vi "lab8.1.vi"() -> ()   [LabVIEW 2018]
panel:
  out "#":dbl
  in  "SELECTOR":sgl(knob) scale=0.0..2.0 scale format="%#_1g"
  out "#3":dbl format="%#_1g"
  out "#2":dbl format="%#_1g"
  out "#1":dbl format="%#_1g"
  in  "PRESS TO\nROLL":bool
  out "output\nnumber":dbl
  in  "toggle":bool
  # "10 & 20\nTOGGLE"
  # "RANDOM #\nGEN"
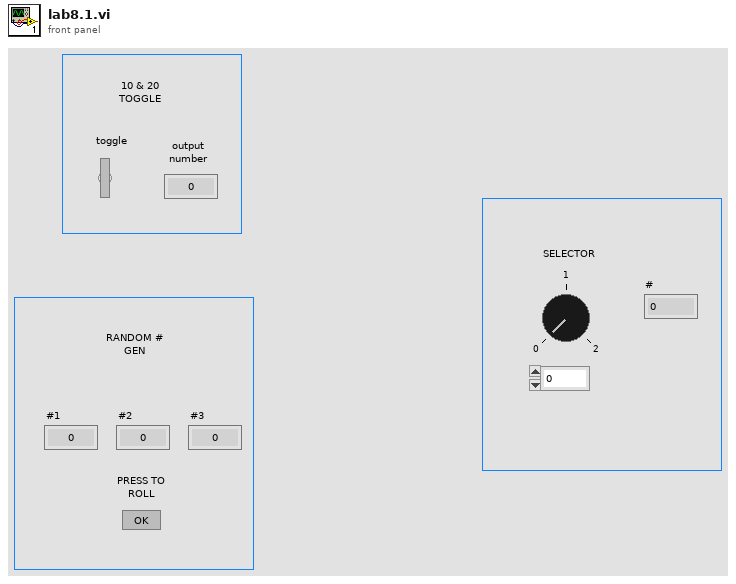
[diagram p1: front panel]
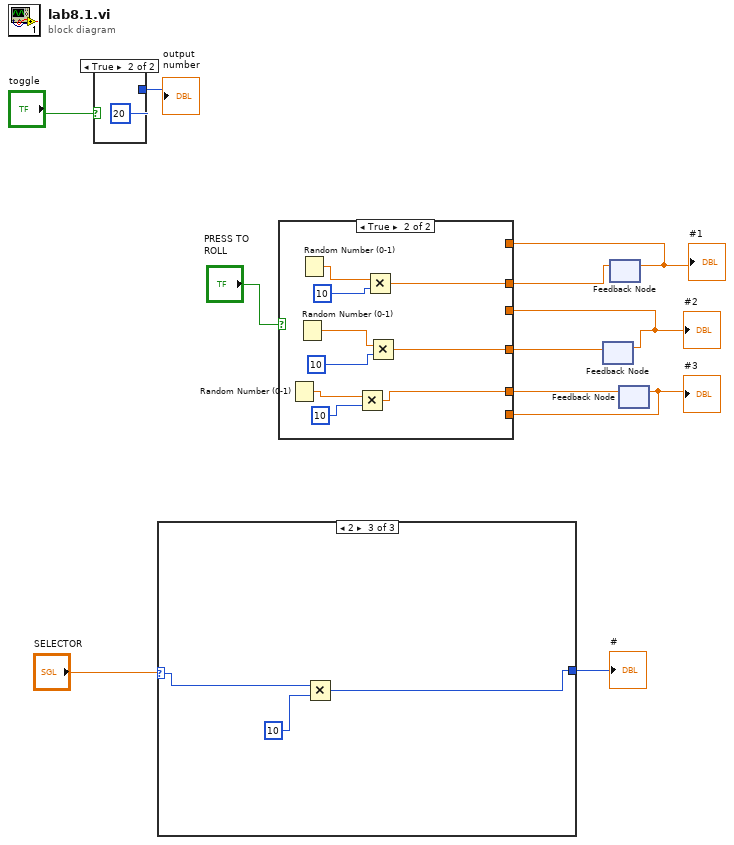
[diagram p0: block diagram]
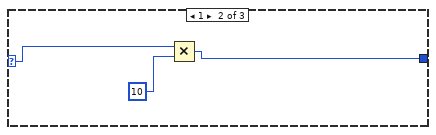
[diagram p3: hidden frame]
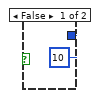
[diagram p5: hidden frame]
diagram:
  n1 = case shown="True" "toggle" {
    tunnel: [10 20] -> w10
    frame False {
    }
    frame True {
    }
  }
  "output\nnumber" <- w10
  n2 = case shown="2" "SELECTOR" {
    selector: "SELECTOR" -> [w14 w16 w19]
    tunnel: [w14 w15 w18] -> w1
    frame 0, Default {
    }
    frame 1 {
      n3 = Multiply(x=w16, y=10) -> (x*y=w15:i32)
    }
    frame 2 {
      n4 = Multiply(x=w19, y=10) -> (x*y=w18:i32)
    }
  }
  "#" <- w1
  n5 = feedback #1() -> (w5:dbl)  [unwired: 1 in]
  "#2" <- w5
  n6 = feedback #2() -> (w6:dbl)  [unwired: 1 in]
  "#1" <- w6
  n7 = feedback #3() -> (w4:dbl)  [unwired: 1 in]
  "#3" <- w4
  n8 = case shown="True" "PRESS TO\nROLL" {
    tunnel: [w23 w26] -> w9
    tunnel: [w22 w25] -> w8
    tunnel: [w21 w24] -> w7
    tunnel: w6 -> [w23 _]
    tunnel: w5 -> [w22 _]
    tunnel: w4 -> [w21 _]
    frame False {
    }
    frame True {
      n9 = Random Number (0-1)() -> (number: 0 to 1=w28:dbl)
      n10 = Random Number (0-1)() -> (number: 0 to 1=w30:dbl)
      n11 = Random Number (0-1)() -> (number: 0 to 1=w32:dbl)
      n12 = Multiply(x=w28, y=10) -> (x*y=w24:dbl)
      n13 = Multiply(x=w32, y=10) -> (x*y=w26:dbl)
      n14 = Multiply(x=w30, y=10) -> (x*y=w25:dbl)
    }
  }
  n15 = feedback-in #1(w8) -> ()
  n16 = feedback-in #2(w9) -> ()
  n17 = feedback-in #3(w7) -> ()
